vi "Write Numeric A.vi"(8 "error in (no error)":errorcluster, 10 "Abs_Integer.lvclass":refnum<class "Abs_Integer.lvclass">, 11 "Divide_Int in":refnum<class "Divide_INT.lvclass">) -> (0 "error out":errorcluster, 3 "Divide_Int out":refnum<class "Divide_INT.lvclass">)   [LabVIEW 2021, in "Divide_INT.lvclass"]
uses:
  Divide_INT.lvclass
  Abs_Types/Integer/Abs_Integer.lvclass
  Divide_INT.lvclass/Divide_INT.ctl
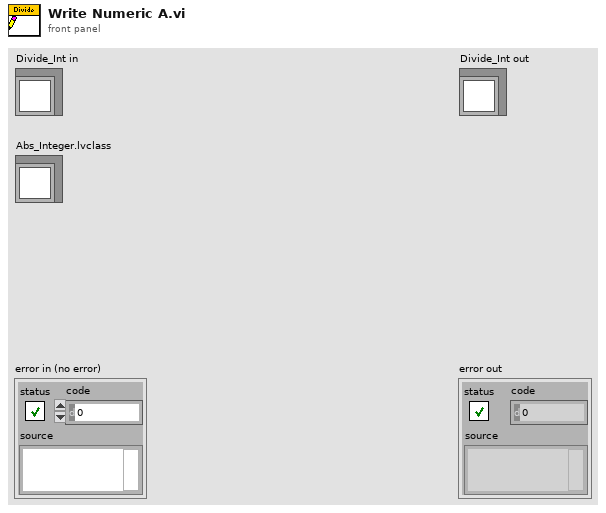
[diagram p1: front panel]
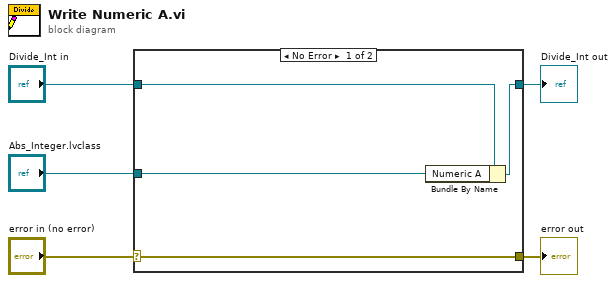
[diagram p0: block diagram]
diagram:
  n1 = case shown="No Error" "error in (no error)" {
    selector: "error in (no error)" -> [w9 w10]
    tunnel: [w9 w10] -> w4
    tunnel: [w7 w11] -> w2
    tunnel: "Divide_Int in" -> [w8 w11]
    tunnel: "Abs_Integer.lvclass" -> [w6 _]
    frame No Error {
      n2 = Bundle By Name(cluster=w8, "Numeric A"=w6) -> (w7:refnum<class "Divide_INT.lvclass">)
    }
    frame Error {
    }
  }
  "error out" <- w4
  "Divide_Int out" <- w2
